vi "Create_Empty_Rx_Channels.vi"(8 "Nb Channels":i32=16, 11 "Rx Channels In":T1[](array[typedef])=[{"Labels Settings"=[{"Name"="label 1", "xmlName"="100", "Label"=23, "transferPeriod"=0, "Driver Data"={"Lbl Tx Hdl"=0, "Decimation"=0, "IterationOffset"=0, "transfer handle"=0, "RX Word"=0, "TXChange"=FALSE, "RX timestamp"=0.0}, "SDI_Enabled"=FALSE, "SDI"=0, "Words"=[{"Block Data Refs"=[], "Values Array"=[0.0], "Length"=1, "FIFO Index"=0, "Param Setting"={"Start Bit"=[10], "Num Bits"=[19], "Signed?"=[FALSE], "ScaleFac"=[1.0], "ScaleOffset"=[0.0], "Channel FIFO Buffer Index"=[1, 0], "Encoding"=[]}}], "bufferSize"=0, "RxWordIdx"=0, "TxWordIdx"=0, "TransferType"=enum."ScheduledLabel", "has timestamp?"=TRUE, "LBL Disable Index"=-1, "Message Handle"=0, "Initialized?"=FALSE}, {"Name"="label 2", "xmlName"="200", "Label"=24, "transferPeriod"=0, "Driver Data"={"Lbl Tx Hdl"=0, "Decimation"=0, "IterationOffset"=0, "transfer handle"=0, "RX Word"=0, "TXChange"=FALSE, "RX timestamp"=0.0}, "SDI_Enabled"=FALSE, "SDI"=0, "Words"=[{"Block Data Refs"=[], "Values Array"=[0.0], "Length"=1, "FIFO Index"=0, "Param Setting"={"Start Bit"=[10], "Num Bits"=[19], "Signed?"=[FALSE], "ScaleFac"=[1.0], "ScaleOffset"=[0.0], "Channel FIFO Buffer Index"=[3, 2], "Encoding"=[]}}], "bufferSize"=0, "RxWordIdx"=0, "TxWordIdx"=0, "TransferType"=enum."ScheduledLabel", "has timestamp?"=TRUE, "LBL Disable Index"=-1, "Message Handle"=0, "Initialized?"=FALSE}, {"Name"="label 3", "xmlName"="300", "Label"=25, "transferPeriod"=0, "Driver Data"={"Lbl Tx Hdl"=0, "Decimation"=0, "IterationOffset"=0, "transfer handle"=0, "RX Word"=0, "TXChange"=FALSE, "RX timestamp"=0.0}, "SDI_Enabled"=FALSE, "SDI"=0, "Words"=[{"Block Data Refs"=[], "Values Array"=[0.0], "Length"=1, "FIFO Index"=0, "Param Setting"={"Start Bit"=[10], "Num Bits"=[19], "Signed?"=[FALSE], "ScaleFac"=[1.0], "ScaleOffset"=[0.0], "Channel FIFO Buffer Index"=[5, 4], "Encoding"=[]}}], "bufferSize"=0, "RxWordIdx"=0, "TxWordIdx"=0, "TransferType"=enum."ScheduledLabel", "has timestamp?"=TRUE, "LBL Disable Index"=-1, "Message Handle"=0, "Initialized?"=FALSE}, {"Name"="label 4", "xmlName"="400", "Label"=26, "transferPeriod"=0, "Driver Data"={"Lbl Tx Hdl"=0, "Decimation"=0, "IterationOffset"=0, "transfer handle"=0, "RX Word"=0, "TXChange"=FALSE, "RX timestamp"=0.0}, "SDI_Enabled"=FALSE, "SDI"=0, "Words"=[{"Block Data Refs"=[], "Values Array"=[0.0], "Length"=1, "FIFO Index"=0, "Param Setting"={"Start Bit"=[10], "Num Bits"=[19], "Signed?"=[FALSE], "ScaleFac"=[1.0], "ScaleOffset"=[0.0], "Channel FIFO Buffer Index"=[7, 6], "Encoding"=[]}}], "bufferSize"=0, "RxWordIdx"=0, "TxWordIdx"=0, "TransferType"=enum."ScheduledLabel", "has timestamp?"=TRUE, "LBL Disable Index"=-1, "Message Handle"=0, "Initialized?"=FALSE}], "channel handle"=0, "channel #"=0, "Label Map"=[], "Label Buffer"=[], "rdBufHandle"=0}, {"Labels Settings"=[{"Name"="label 1", "xmlName"="101", "Label"=23, "transferPeriod"=0, "Driver Data"={"Lbl Tx Hdl"=0, "Decimation"=0, "IterationOffset"=0, "transfer handle"=0, "RX Word"=0, "TXChange"=FALSE, "RX timestamp"=0.0}, "SDI_Enabled"=FALSE, "SDI"=0, "Words"=[{"Block Data Refs"=[], "Values Array"=[0.0], "Length"=1, "FIFO Index"=0, "Param Setting"={"Start Bit"=[10], "Num Bits"=[19], "Signed?"=[FALSE], "ScaleFac"=[1.0], "ScaleOffset"=[0.0], "Channel FIFO Buffer Index"=[9, 8], "Encoding"=[]}}], "bufferSize"=0, "RxWordIdx"=0, "TxWordIdx"=0, "TransferType"=enum."ScheduledLabel", "has timestamp?"=TRUE, "LBL Disable Index"=-1, "Message Handle"=0, "Initialized?"=FALSE}, {"Name"="label 2", "xmlName"="201", "Label"=24, "transferPeriod"=0, "Driver Data"={"Lbl Tx Hdl"=0, "Decimation"=0, "IterationOffset"=0, "transfer handle"=0, "RX Word"=0, "TXChange"=FALSE, "RX timestamp"=0.0}, "SDI_Enabled"=FALSE, "SDI"=0, "Words"=[{"Block Data Refs"=[], "Values Array"=[0.0], "Length"=1, "FIFO Index"=0, "Param Setting"={"Start Bit"=[10], "Num Bits"=[19], "Signed?"=[FALSE], "ScaleFac"=[1.0], "ScaleOffset"=[0.0], "Channel FIFO Buffer Index"=[11, 10], "Encoding"=[]}}], "bufferSize"=0, "RxWordIdx"=0, "TxWordIdx"=0, "TransferType"=enum."ScheduledLabel", "has timestamp?"=TRUE, "LBL Disable Index"=-1, "Message Handle"=0, "Initialized?"=FALSE}, {"Name"="label 3", "xmlName"="301", "Label"=25, "transferPeriod"=0, "Driver Data"={"Lbl Tx Hdl"=0, "Decimation"=0, "IterationOffset"=0, "transfer handle"=0, "RX Word"=0, "TXChange"=FALSE, "RX timestamp"=0.0}, "SDI_Enabled"=FALSE, "SDI"=0, "Words"=[{"Block Data Refs"=[], "Values Array"=[0.0], "Length"=1, "FIFO Index"=0, "Param Setting"={"Start Bit"=[10], "Num Bits"=[19], "Signed?"=[FALSE], "ScaleFac"=[1.0], "ScaleOffset"=[0.0], "Channel FIFO Buffer Index"=[13, 12], "Encoding"=[]}}], "bufferSize"=0, "RxWordIdx"=0, "TxWordIdx"=0, "TransferType"=enum."ScheduledLabel", "has timestamp?"=TRUE, "LBL Disable Index"=-1, "Message Handle"=0, "Initialized?"=FALSE}, {"Name"="label 4", "xmlName"="401", "Label"=26, "transferPeriod"=0, "Driver Data"={"Lbl Tx Hdl"=0, "Decimation"=0, "IterationOffset"=0, "transfer handle"=0, "RX Word"=0, "TXChange"=FALSE, "RX timestamp"=0.0}, "SDI_Enabled"=FALSE, "SDI"=0, "Words"=[{"Block Data Refs"=[], "Values Array"=[0.0], "Length"=1, "FIFO Index"=0, "Param Setting"={"Start Bit"=[10], "Num Bits"=[19], "Signed?"=[FALSE], "ScaleFac"=[1.0], "ScaleOffset"=[0.0], "Channel FIFO Buffer Index"=[15, 14], "Encoding"=[]}}], "bufferSize"=0, "RxWordIdx"=0, "TxWordIdx"=0, "TransferType"=enum."ScheduledLabel", "has timestamp?"=TRUE, "LBL Disable Index"=-1, "Message Handle"=0, "Initialized?"=FALSE}, {"Name"="label 5", "xmlName"="501", "Label"=27, "transferPeriod"=0, "Driver Data"={"Lbl Tx Hdl"=0, "Decimation"=0, "IterationOffset"=0, "transfer handle"=0, "RX Word"=0, "TXChange"=FALSE, "RX timestamp"=0.0}, "SDI_Enabled"=FALSE, "SDI"=0, "Words"=[{"Block Data Refs"=[], "Values Array"=[0.0], "Length"=1, "FIFO Index"=0, "Param Setting"={"Start Bit"=[10], "Num Bits"=[19], "Signed?"=[FALSE], "ScaleFac"=[1.0], "ScaleOffset"=[0.0], "Channel FIFO Buffer Index"=[17, 16], "Encoding"=[]}}], "bufferSize"=0, "RxWordIdx"=0, "TxWordIdx"=0, "TransferType"=enum."ScheduledLabel", "has timestamp?"=TRUE, "LBL Disable Index"=-1, "Message Handle"=0, "Initialized?"=FALSE}, {"Name"="label 6", "xmlName"="601", "Label"=28, "transferPeriod"=0, "Driver Data"={"Lbl Tx Hdl"=0, "Decimation"=0, "IterationOffset"=0, "transfer handle"=0, "RX Word"=0, "TXChange"=FALSE, "RX timestamp"=0.0}, "SDI_Enabled"=FALSE, "SDI"=0, "Words"=[{"Block Data Refs"=[], "Values Array"=[0.0], "Length"=1, "FIFO Index"=0, "Param Setting"={"Start Bit"=[10], "Num Bits"=[19], "Signed?"=[FALSE], "ScaleFac"=[1.0], "ScaleOffset"=[0.0], "Channel FIFO Buffer Index"=[19, 18], "Encoding"=[]}}], "bufferSize"=0, "RxWordIdx"=0, "TxWordIdx"=0, "TransferType"=enum."ScheduledLabel", "has timestamp?"=TRUE, "LBL Disable Index"=-1, "Message Handle"=0, "Initialized?"=FALSE}], "channel handle"=0, "channel #"=1, "Label Map"=[], "Label Buffer"=[], "rdBufHandle"=0}, {"Labels Settings"=[{"Name"="label 1", "xmlName"="102", "Label"=23, "transferPeriod"=0, "Driver Data"={"Lbl Tx Hdl"=0, "Decimation"=0, "IterationOffset"=0, "transfer handle"=0, "RX Word"=0, "TXChange"=FALSE, "RX timestamp"=0.0}, "SDI_Enabled"=FALSE, "SDI"=0, "Words"=[{"Block Data Refs"=[], "Values Array"=[0.0], "Length"=1, "FIFO Index"=0, "Param Setting"={"Start Bit"=[10], "Num Bits"=[19], "Signed?"=[FALSE], "ScaleFac"=[1.0], "ScaleOffset"=[0.0], "Channel FIFO Buffer Index"=[21, 20], "Encoding"=[]}}], "bufferSize"=0, "RxWordIdx"=0, "TxWordIdx"=0, "TransferType"=enum."ScheduledLabel", "has timestamp?"=TRUE, "LBL Disable Index"=-1, "Message Handle"=0, "Initialized?"=FALSE}, {"Name"="label 2", "xmlName"="202", "Label"=24, "transferPeriod"=0, "Driver Data"={"Lbl Tx Hdl"=0, "Decimation"=0, "IterationOffset"=0, "transfer handle"=0, "RX Word"=0, "TXChange"=FALSE, "RX timestamp"=0.0}, "SDI_Enabled"=FALSE, "SDI"=0, "Words"=[{"Block Data Refs"=[], "Values Array"=[0.0], "Length"=1, "FIFO Index"=0, "Param Setting"={"Start Bit"=[10], "Num Bits"=[19], "Signed?"=[FALSE], "ScaleFac"=[1.0], "ScaleOffset"=[0.0], "Channel FIFO Buffer Index"=[23, 22], "Encoding"=[]}}], "bufferSize"=0, "RxWordIdx"=0, "TxWordIdx"=0, "TransferType"=enum."ScheduledLabel", "has timestamp?"=TRUE, "LBL Disable Index"=-1, "Message Handle"=0, "Initialized?"=FALSE}, {"Name"="label 3", "xmlName"="302", "Label"=25, "transferPeriod"=0, "Driver Data"={"Lbl Tx Hdl"=0, "Decimation"=0, "IterationOffset"=0, "transfer handle"=0, "RX Word"=0, "TXChange"=FALSE, "RX timestamp"=0.0}, "SDI_Enabled"=FALSE, "SDI"=0, "Words"=[{"Block Data Refs"=[], "Values Array"=[0.0], "Length"=1, "FIFO Index"=0, "Param Setting"={"Start Bit"=[10], "Num Bits"=[19], "Signed?"=[FALSE], "ScaleFac"=[1.0], "ScaleOffset"=[0.0], "Channel FIFO Buffer Index"=[25, 24], "Encoding"=[]}}], "bufferSize"=0, "RxWordIdx"=0, "TxWordIdx"=0, "TransferType"=enum."ScheduledLabel", "has timestamp?"=TRUE, "LBL Disable Index"=-1, "Message Handle"=0, "Initialized?"=FALSE}, {"Name"="label 4", "xmlName"="402", "Label"=26, "transferPeriod"=0, "Driver Data"={"Lbl Tx Hdl"=0, "Decimation"=0, "IterationOffset"=0, "transfer handle"=0, "RX Word"=0, "TXChange"=FALSE, "RX timestamp"=0.0}, "SDI_Enabled"=FALSE, "SDI"=0, "Words"=[{"Block Data Refs"=[], "Values Array"=[0.0], "Length"=1, "FIFO Index"=0, "Param Setting"={"Start Bit"=[10], "Num Bits"=[19], "Signed?"=[FALSE], "ScaleFac"=[1.0], "ScaleOffset"=[0.0], "Channel FIFO Buffer Index"=[27, 26], "Encoding"=[]}}], "bufferSize"=0, "RxWordIdx"=0, "TxWordIdx"=0, "TransferType"=enum."ScheduledLabel", "has timestamp?"=TRUE, "LBL Disable Index"=-1, "Message Handle"=0, "Initialized?"=FALSE}, {"Name"="label 5", "xmlName"="502", "Label"=27, "transferPeriod"=0, "Driver Data"={"Lbl Tx Hdl"=0, "Decimation"=0, "IterationOffset"=0, "transfer handle"=0, "RX Word"=0, "TXChange"=FALSE, "RX timestamp"=0.0}, "SDI_Enabled"=FALSE, "SDI"=0, "Words"=[{"Block Data Refs"=[], "Values Array"=[0.0], "Length"=1, "FIFO Index"=0, "Param Setting"={"Start Bit"=[10], "Num Bits"=[19], "Signed?"=[FALSE], "ScaleFac"=[1.0], "ScaleOffset"=[0.0], "Channel FIFO Buffer Index"=[28, 29], "Encoding"=[]}}], "bufferSize"=0, "RxWordIdx"=0, "TxWordIdx"=0, "TransferType"=enum."ScheduledLabel", "has timestamp?"=TRUE, "LBL Disable Index"=-1, "Message Handle"=0, "Initialized?"=FALSE}, {"Name"="label 6", "xmlName"="602", "Label"=28, "transferPeriod"=0, "Driver Data"={"Lbl Tx Hdl"=0, "Decimation"=0, "IterationOffset"=0, "transfer handle"=0, "RX Word"=0, "TXChange"=FALSE, "RX timestamp"=0.0}, "SDI_Enabled"=FALSE, "SDI"=0, "Words"=[{"Block Data Refs"=[], "Values Array"=[0.0], "Length"=1, "FIFO Index"=0, "Param Setting"={"Start Bit"=[10], "Num Bits"=[19], "Signed?"=[FALSE], "ScaleFac"=[1.0], "ScaleOffset"=[0.0], "Channel FIFO Buffer Index"=[31, 30], "Encoding"=[]}}], "bufferSize"=0, "RxWordIdx"=0, "TxWordIdx"=0, "TransferType"=enum."ScheduledLabel", "has timestamp?"=TRUE, "LBL Disable Index"=-1, "Message Handle"=0, "Initialized?"=FALSE}, {"Name"="label 7", "xmlName"="702", "Label"=29, "transferPeriod"=0, "Driver Data"={"Lbl Tx Hdl"=0, "Decimation"=0, "IterationOffset"=0, "transfer handle"=0, "RX Word"=0, "TXChange"=FALSE, "RX timestamp"=0.0}, "SDI_Enabled"=FALSE, "SDI"=0, "Words"=[{"Block Data Refs"=[], "Values Array"=[0.0], "Length"=1, "FIFO Index"=0, "Param Setting"={"Start Bit"=[10], "Num Bits"=[19], "Signed?"=[FALSE], "ScaleFac"=[1.0], "ScaleOffset"=[0.0], "Channel FIFO Buffer Index"=[33, 32], "Encoding"=[]}}], "bufferSize"=0, "RxWordIdx"=0, "TxWordIdx"=0, "TransferType"=enum."ScheduledLabel", "has timestamp?"=TRUE, "LBL Disable Index"=-1, "Message Handle"=0, "Initialized?"=FALSE}, {"Name"="label 8", "xmlName"="802", "Label"=30, "transferPeriod"=0, "Driver Data"={"Lbl Tx Hdl"=0, "Decimation"=0, "IterationOffset"=0, "transfer handle"=0, "RX Word"=0, "TXChange"=FALSE, "RX timestamp"=0.0}, "SDI_Enabled"=FALSE, "SDI"=0, "Words"=[{"Block Data Refs"=[], "Values Array"=[0.0], "Length"=1, "FIFO Index"=0, "Param Setting"={"Start Bit"=[10], "Num Bits"=[19], "Signed?"=[FALSE], "ScaleFac"=[1.0], "ScaleOffset"=[0.0], "Channel FIFO Buffer Index"=[35, 34], "Encoding"=[]}}], "bufferSize"=0, "RxWordIdx"=0, "TxWordIdx"=0, "TransferType"=enum."ScheduledLabel", "has timestamp?"=TRUE, "LBL Disable Index"=-1, "Message Handle"=0, "Initialized?"=FALSE}], "channel handle"=0, "channel #"=2, "Label Map"=[], "Label Buffer"=[], "rdBufHandle"=0}, {"Labels Settings"=[{"Name"="label 1 SDI 01", "xmlName"="10301", "Label"=23, "transferPeriod"=0, "Driver Data"={"Lbl Tx Hdl"=0, "Decimation"=0, "IterationOffset"=0, "transfer handle"=0, "RX Word"=0, "TXChange"=FALSE, "RX timestamp"=0.0}, "SDI_Enabled"=TRUE, "SDI"=1, "Words"=[{"Block Data Refs"=[], "Values Array"=[0.0], "Length"=1, "FIFO Index"=0, "Param Setting"={"Start Bit"=[10], "Num Bits"=[19], "Signed?"=[FALSE], "ScaleFac"=[1.0], "ScaleOffset"=[0.0], "Channel FIFO Buffer Index"=[37, 36], "Encoding"=[]}}], "bufferSize"=0, "RxWordIdx"=0, "TxWordIdx"=0, "TransferType"=enum."ScheduledLabel", "has timestamp?"=TRUE, "LBL Disable Index"=-1, "Message Handle"=0, "Initialized?"=FALSE}, {"Name"="label 1 SDI 10", "xmlName"="10310", "Label"=23, "transferPeriod"=0, "Driver Data"={"Lbl Tx Hdl"=0, "Decimation"=0, "IterationOffset"=0, "transfer handle"=0, "RX Word"=0, "TXChange"=FALSE, "RX timestamp"=0.0}, "SDI_Enabled"=TRUE, "SDI"=10, "Words"=[{"Block Data Refs"=[], "Values Array"=[0.0], "Length"=1, "FIFO Index"=0, "Param Setting"={"Start Bit"=[10], "Num Bits"=[19], "Signed?"=[FALSE], "ScaleFac"=[1.0], "ScaleOffset"=[0.0], "Channel FIFO Buffer Index"=[39, 38], "Encoding"=[]}}], "bufferSize"=0, "RxWordIdx"=0, "TxWordIdx"=0, "TransferType"=enum."ScheduledLabel", "has timestamp?"=TRUE, "LBL Disable Index"=-1, "Message Handle"=0, "Initialized?"=FALSE}, {"Name"="label 2", "xmlName"="203", "Label"=24, "transferPeriod"=0, "Driver Data"={"Lbl Tx Hdl"=0, "Decimation"=0, "IterationOffset"=0, "transfer handle"=0, "RX Word"=0, "TXChange"=FALSE, "RX timestamp"=0.0}, "SDI_Enabled"=FALSE, "SDI"=0, "Words"=[{"Block Data Refs"=[], "Values Array"=[0.0], "Length"=1, "FIFO Index"=0, "Param Setting"={"Start Bit"=[10], "Num Bits"=[19], "Signed?"=[FALSE], "ScaleFac"=[1.0], "ScaleOffset"=[0.0], "Channel FIFO Buffer Index"=[41, 40], "Encoding"=[]}}], "bufferSize"=0, "RxWordIdx"=0, "TxWordIdx"=0, "TransferType"=enum."ScheduledLabel", "has timestamp?"=TRUE, "LBL Disable Index"=-1, "Message Handle"=0, "Initialized?"=FALSE}], "channel handle"=0, "channel #"=3, "Label Map"=[], "Label Buffer"=[], "rdBufHandle"=0}] {"Labels Settings"."Label" format="%.0o"}) -> (3 "Rx Channels Out":T1[](array[typedef])=[{"Labels Settings"=[{"Name"="label 1", "xmlName"="100", "Label"=23, "transferPeriod"=0, "Driver Data"={"Lbl Tx Hdl"=0, "Decimation"=0, "IterationOffset"=0, "transfer handle"=0, "RX Word"=0, "TXChange"=FALSE, "RX timestamp"=0.0}, "SDI_Enabled"=FALSE, "SDI"=0, "Words"=[{"Block Data Refs"=[], "Values Array"=[0.0], "Length"=1, "FIFO Index"=0, "Param Setting"={"Start Bit"=[10], "Num Bits"=[19], "Signed?"=[FALSE], "ScaleFac"=[1.0], "ScaleOffset"=[0.0], "Channel FIFO Buffer Index"=[1, 0], "Encoding"=[]}}], "bufferSize"=0, "RxWordIdx"=0, "TxWordIdx"=0, "TransferType"=enum."ScheduledLabel", "has timestamp?"=TRUE, "LBL Disable Index"=-1, "Message Handle"=0, "Initialized?"=FALSE}, {"Name"="label 2", "xmlName"="200", "Label"=24, "transferPeriod"=0, "Driver Data"={"Lbl Tx Hdl"=0, "Decimation"=0, "IterationOffset"=0, "transfer handle"=0, "RX Word"=0, "TXChange"=FALSE, "RX timestamp"=0.0}, "SDI_Enabled"=FALSE, "SDI"=0, "Words"=[{"Block Data Refs"=[], "Values Array"=[0.0], "Length"=1, "FIFO Index"=0, "Param Setting"={"Start Bit"=[10], "Num Bits"=[19], "Signed?"=[FALSE], "ScaleFac"=[1.0], "ScaleOffset"=[0.0], "Channel FIFO Buffer Index"=[3, 2], "Encoding"=[]}}], "bufferSize"=0, "RxWordIdx"=0, "TxWordIdx"=0, "TransferType"=enum."ScheduledLabel", "has timestamp?"=TRUE, "LBL Disable Index"=-1, "Message Handle"=0, "Initialized?"=FALSE}, {"Name"="label 3", "xmlName"="300", "Label"=25, "transferPeriod"=0, "Driver Data"={"Lbl Tx Hdl"=0, "Decimation"=0, "IterationOffset"=0, "transfer handle"=0, "RX Word"=0, "TXChange"=FALSE, "RX timestamp"=0.0}, "SDI_Enabled"=FALSE, "SDI"=0, "Words"=[{"Block Data Refs"=[], "Values Array"=[0.0], "Length"=1, "FIFO Index"=0, "Param Setting"={"Start Bit"=[10], "Num Bits"=[19], "Signed?"=[FALSE], "ScaleFac"=[1.0], "ScaleOffset"=[0.0], "Channel FIFO Buffer Index"=[5, 4], "Encoding"=[]}}], "bufferSize"=0, "RxWordIdx"=0, "TxWordIdx"=0, "TransferType"=enum."ScheduledLabel", "has timestamp?"=TRUE, "LBL Disable Index"=-1, "Message Handle"=0, "Initialized?"=FALSE}, {"Name"="label 4", "xmlName"="400", "Label"=26, "transferPeriod"=0, "Driver Data"={"Lbl Tx Hdl"=0, "Decimation"=0, "IterationOffset"=0, "transfer handle"=0, "RX Word"=0, "TXChange"=FALSE, "RX timestamp"=0.0}, "SDI_Enabled"=FALSE, "SDI"=0, "Words"=[{"Block Data Refs"=[], "Values Array"=[0.0], "Length"=1, "FIFO Index"=0, "Param Setting"={"Start Bit"=[10], "Num Bits"=[19], "Signed?"=[FALSE], "ScaleFac"=[1.0], "ScaleOffset"=[0.0], "Channel FIFO Buffer Index"=[7, 6], "Encoding"=[]}}], "bufferSize"=0, "RxWordIdx"=0, "TxWordIdx"=0, "TransferType"=enum."ScheduledLabel", "has timestamp?"=TRUE, "LBL Disable Index"=-1, "Message Handle"=0, "Initialized?"=FALSE}], "channel handle"=0, "channel #"=0, "Label Map"=[], "Label Buffer"=[], "rdBufHandle"=0}, {"Labels Settings"=[{"Name"="label 1", "xmlName"="101", "Label"=23, "transferPeriod"=0, "Driver Data"={"Lbl Tx Hdl"=0, "Decimation"=0, "IterationOffset"=0, "transfer handle"=0, "RX Word"=0, "TXChange"=FALSE, "RX timestamp"=0.0}, "SDI_Enabled"=FALSE, "SDI"=0, "Words"=[{"Block Data Refs"=[], "Values Array"=[0.0], "Length"=1, "FIFO Index"=0, "Param Setting"={"Start Bit"=[10], "Num Bits"=[19], "Signed?"=[FALSE], "ScaleFac"=[1.0], "ScaleOffset"=[0.0], "Channel FIFO Buffer Index"=[9, 8], "Encoding"=[]}}], "bufferSize"=0, "RxWordIdx"=0, "TxWordIdx"=0, "TransferType"=enum."ScheduledLabel", "has timestamp?"=TRUE, "LBL Disable Index"=-1, "Message Handle"=0, "Initialized?"=FALSE}, {"Name"="label 2", "xmlName"="201", "Label"=24, "transferPeriod"=0, "Driver Data"={"Lbl Tx Hdl"=0, "Decimation"=0, "IterationOffset"=0, "transfer handle"=0, "RX Word"=0, "TXChange"=FALSE, "RX timestamp"=0.0}, "SDI_Enabled"=FALSE, "SDI"=0, "Words"=[{"Block Data Refs"=[], "Values Array"=[0.0], "Length"=1, "FIFO Index"=0, "Param Setting"={"Start Bit"=[10], "Num Bits"=[19], "Signed?"=[FALSE], "ScaleFac"=[1.0], "ScaleOffset"=[0.0], "Channel FIFO Buffer Index"=[11, 10], "Encoding"=[]}}], "bufferSize"=0, "RxWordIdx"=0, "TxWordIdx"=0, "TransferType"=enum."ScheduledLabel", "has timestamp?"=TRUE, "LBL Disable Index"=-1, "Message Handle"=0, "Initialized?"=FALSE}, {"Name"="label 3", "xmlName"="301", "Label"=25, "transferPeriod"=0, "Driver Data"={"Lbl Tx Hdl"=0, "Decimation"=0, "IterationOffset"=0, "transfer handle"=0, "RX Word"=0, "TXChange"=FALSE, "RX timestamp"=0.0}, "SDI_Enabled"=FALSE, "SDI"=0, "Words"=[{"Block Data Refs"=[], "Values Array"=[0.0], "Length"=1, "FIFO Index"=0, "Param Setting"={"Start Bit"=[10], "Num Bits"=[19], "Signed?"=[FALSE], "ScaleFac"=[1.0], "ScaleOffset"=[0.0], "Channel FIFO Buffer Index"=[13, 12], "Encoding"=[]}}], "bufferSize"=0, "RxWordIdx"=0, "TxWordIdx"=0, "TransferType"=enum."ScheduledLabel", "has timestamp?"=TRUE, "LBL Disable Index"=-1, "Message Handle"=0, "Initialized?"=FALSE}, {"Name"="label 4", "xmlName"="401", "Label"=26, "transferPeriod"=0, "Driver Data"={"Lbl Tx Hdl"=0, "Decimation"=0, "IterationOffset"=0, "transfer handle"=0, "RX Word"=0, "TXChange"=FALSE, "RX timestamp"=0.0}, "SDI_Enabled"=FALSE, "SDI"=0, "Words"=[{"Block Data Refs"=[], "Values Array"=[0.0], "Length"=1, "FIFO Index"=0, "Param Setting"={"Start Bit"=[10], "Num Bits"=[19], "Signed?"=[FALSE], "ScaleFac"=[1.0], "ScaleOffset"=[0.0], "Channel FIFO Buffer Index"=[15, 14], "Encoding"=[]}}], "bufferSize"=0, "RxWordIdx"=0, "TxWordIdx"=0, "TransferType"=enum."ScheduledLabel", "has timestamp?"=TRUE, "LBL Disable Index"=-1, "Message Handle"=0, "Initialized?"=FALSE}, {"Name"="label 5", "xmlName"="501", "Label"=27, "transferPeriod"=0, "Driver Data"={"Lbl Tx Hdl"=0, "Decimation"=0, "IterationOffset"=0, "transfer handle"=0, "RX Word"=0, "TXChange"=FALSE, "RX timestamp"=0.0}, "SDI_Enabled"=FALSE, "SDI"=0, "Words"=[{"Block Data Refs"=[], "Values Array"=[0.0], "Length"=1, "FIFO Index"=0, "Param Setting"={"Start Bit"=[10], "Num Bits"=[19], "Signed?"=[FALSE], "ScaleFac"=[1.0], "ScaleOffset"=[0.0], "Channel FIFO Buffer Index"=[17, 16], "Encoding"=[]}}], "bufferSize"=0, "RxWordIdx"=0, "TxWordIdx"=0, "TransferType"=enum."ScheduledLabel", "has timestamp?"=TRUE, "LBL Disable Index"=-1, "Message Handle"=0, "Initialized?"=FALSE}, {"Name"="label 6", "xmlName"="601", "Label"=28, "transferPeriod"=0, "Driver Data"={"Lbl Tx Hdl"=0, "Decimation"=0, "IterationOffset"=0, "transfer handle"=0, "RX Word"=0, "TXChange"=FALSE, "RX timestamp"=0.0}, "SDI_Enabled"=FALSE, "SDI"=0, "Words"=[{"Block Data Refs"=[], "Values Array"=[0.0], "Length"=1, "FIFO Index"=0, "Param Setting"={"Start Bit"=[10], "Num Bits"=[19], "Signed?"=[FALSE], "ScaleFac"=[1.0], "ScaleOffset"=[0.0], "Channel FIFO Buffer Index"=[19, 18], "Encoding"=[]}}], "bufferSize"=0, "RxWordIdx"=0, "TxWordIdx"=0, "TransferType"=enum."ScheduledLabel", "has timestamp?"=TRUE, "LBL Disable Index"=-1, "Message Handle"=0, "Initialized?"=FALSE}], "channel handle"=0, "channel #"=1, "Label Map"=[], "Label Buffer"=[], "rdBufHandle"=0}, {"Labels Settings"=[{"Name"="label 1", "xmlName"="102", "Label"=23, "transferPeriod"=0, "Driver Data"={"Lbl Tx Hdl"=0, "Decimation"=0, "IterationOffset"=0, "transfer handle"=0, "RX Word"=0, "TXChange"=FALSE, "RX timestamp"=0.0}, "SDI_Enabled"=FALSE, "SDI"=0, "Words"=[{"Block Data Refs"=[], "Values Array"=[0.0], "Length"=1, "FIFO Index"=0, "Param Setting"={"Start Bit"=[10], "Num Bits"=[19], "Signed?"=[FALSE], "ScaleFac"=[1.0], "ScaleOffset"=[0.0], "Channel FIFO Buffer Index"=[21, 20], "Encoding"=[]}}], "bufferSize"=0, "RxWordIdx"=0, "TxWordIdx"=0, "TransferType"=enum."ScheduledLabel", "has timestamp?"=TRUE, "LBL Disable Index"=-1, "Message Handle"=0, "Initialized?"=FALSE}, {"Name"="label 2", "xmlName"="202", "Label"=24, "transferPeriod"=0, "Driver Data"={"Lbl Tx Hdl"=0, "Decimation"=0, "IterationOffset"=0, "transfer handle"=0, "RX Word"=0, "TXChange"=FALSE, "RX timestamp"=0.0}, "SDI_Enabled"=FALSE, "SDI"=0, "Words"=[{"Block Data Refs"=[], "Values Array"=[0.0], "Length"=1, "FIFO Index"=0, "Param Setting"={"Start Bit"=[10], "Num Bits"=[19], "Signed?"=[FALSE], "ScaleFac"=[1.0], "ScaleOffset"=[0.0], "Channel FIFO Buffer Index"=[23, 22], "Encoding"=[]}}], "bufferSize"=0, "RxWordIdx"=0, "TxWordIdx"=0, "TransferType"=enum."ScheduledLabel", "has timestamp?"=TRUE, "LBL Disable Index"=-1, "Message Handle"=0, "Initialized?"=FALSE}, {"Name"="label 3", "xmlName"="302", "Label"=25, "transferPeriod"=0, "Driver Data"={"Lbl Tx Hdl"=0, "Decimation"=0, "IterationOffset"=0, "transfer handle"=0, "RX Word"=0, "TXChange"=FALSE, "RX timestamp"=0.0}, "SDI_Enabled"=FALSE, "SDI"=0, "Words"=[{"Block Data Refs"=[], "Values Array"=[0.0], "Length"=1, "FIFO Index"=0, "Param Setting"={"Start Bit"=[10], "Num Bits"=[19], "Signed?"=[FALSE], "ScaleFac"=[1.0], "ScaleOffset"=[0.0], "Channel FIFO Buffer Index"=[25, 24], "Encoding"=[]}}], "bufferSize"=0, "RxWordIdx"=0, "TxWordIdx"=0, "TransferType"=enum."ScheduledLabel", "has timestamp?"=TRUE, "LBL Disable Index"=-1, "Message Handle"=0, "Initialized?"=FALSE}, {"Name"="label 4", "xmlName"="402", "Label"=26, "transferPeriod"=0, "Driver Data"={"Lbl Tx Hdl"=0, "Decimation"=0, "IterationOffset"=0, "transfer handle"=0, "RX Word"=0, "TXChange"=FALSE, "RX timestamp"=0.0}, "SDI_Enabled"=FALSE, "SDI"=0, "Words"=[{"Block Data Refs"=[], "Values Array"=[0.0], "Length"=1, "FIFO Index"=0, "Param Setting"={"Start Bit"=[10], "Num Bits"=[19], "Signed?"=[FALSE], "ScaleFac"=[1.0], "ScaleOffset"=[0.0], "Channel FIFO Buffer Index"=[27, 26], "Encoding"=[]}}], "bufferSize"=0, "RxWordIdx"=0, "TxWordIdx"=0, "TransferType"=enum."ScheduledLabel", "has timestamp?"=TRUE, "LBL Disable Index"=-1, "Message Handle"=0, "Initialized?"=FALSE}, {"Name"="label 5", "xmlName"="502", "Label"=27, "transferPeriod"=0, "Driver Data"={"Lbl Tx Hdl"=0, "Decimation"=0, "IterationOffset"=0, "transfer handle"=0, "RX Word"=0, "TXChange"=FALSE, "RX timestamp"=0.0}, "SDI_Enabled"=FALSE, "SDI"=0, "Words"=[{"Block Data Refs"=[], "Values Array"=[0.0], "Length"=1, "FIFO Index"=0, "Param Setting"={"Start Bit"=[10], "Num Bits"=[19], "Signed?"=[FALSE], "ScaleFac"=[1.0], "ScaleOffset"=[0.0], "Channel FIFO Buffer Index"=[28, 29], "Encoding"=[]}}], "bufferSize"=0, "RxWordIdx"=0, "TxWordIdx"=0, "TransferType"=enum."ScheduledLabel", "has timestamp?"=TRUE, "LBL Disable Index"=-1, "Message Handle"=0, "Initialized?"=FALSE}, {"Name"="label 6", "xmlName"="602", "Label"=28, "transferPeriod"=0, "Driver Data"={"Lbl Tx Hdl"=0, "Decimation"=0, "IterationOffset"=0, "transfer handle"=0, "RX Word"=0, "TXChange"=FALSE, "RX timestamp"=0.0}, "SDI_Enabled"=FALSE, "SDI"=0, "Words"=[{"Block Data Refs"=[], "Values Array"=[0.0], "Length"=1, "FIFO Index"=0, "Param Setting"={"Start Bit"=[10], "Num Bits"=[19], "Signed?"=[FALSE], "ScaleFac"=[1.0], "ScaleOffset"=[0.0], "Channel FIFO Buffer Index"=[31, 30], "Encoding"=[]}}], "bufferSize"=0, "RxWordIdx"=0, "TxWordIdx"=0, "TransferType"=enum."ScheduledLabel", "has timestamp?"=TRUE, "LBL Disable Index"=-1, "Message Handle"=0, "Initialized?"=FALSE}, {"Name"="label 7", "xmlName"="702", "Label"=29, "transferPeriod"=0, "Driver Data"={"Lbl Tx Hdl"=0, "Decimation"=0, "IterationOffset"=0, "transfer handle"=0, "RX Word"=0, "TXChange"=FALSE, "RX timestamp"=0.0}, "SDI_Enabled"=FALSE, "SDI"=0, "Words"=[{"Block Data Refs"=[], "Values Array"=[0.0], "Length"=1, "FIFO Index"=0, "Param Setting"={"Start Bit"=[10], "Num Bits"=[19], "Signed?"=[FALSE], "ScaleFac"=[1.0], "ScaleOffset"=[0.0], "Channel FIFO Buffer Index"=[33, 32], "Encoding"=[]}}], "bufferSize"=0, "RxWordIdx"=0, "TxWordIdx"=0, "TransferType"=enum."ScheduledLabel", "has timestamp?"=TRUE, "LBL Disable Index"=-1, "Message Handle"=0, "Initialized?"=FALSE}, {"Name"="label 8", "xmlName"="802", "Label"=30, "transferPeriod"=0, "Driver Data"={"Lbl Tx Hdl"=0, "Decimation"=0, "IterationOffset"=0, "transfer handle"=0, "RX Word"=0, "TXChange"=FALSE, "RX timestamp"=0.0}, "SDI_Enabled"=FALSE, "SDI"=0, "Words"=[{"Block Data Refs"=[], "Values Array"=[0.0], "Length"=1, "FIFO Index"=0, "Param Setting"={"Start Bit"=[10], "Num Bits"=[19], "Signed?"=[FALSE], "ScaleFac"=[1.0], "ScaleOffset"=[0.0], "Channel FIFO Buffer Index"=[35, 34], "Encoding"=[]}}], "bufferSize"=0, "RxWordIdx"=0, "TxWordIdx"=0, "TransferType"=enum."ScheduledLabel", "has timestamp?"=TRUE, "LBL Disable Index"=-1, "Message Handle"=0, "Initialized?"=FALSE}], "channel handle"=0, "channel #"=2, "Label Map"=[], "Label Buffer"=[], "rdBufHandle"=0}, {"Labels Settings"=[{"Name"="label 1 SDI 01", "xmlName"="10301", "Label"=23, "transferPeriod"=0, "Driver Data"={"Lbl Tx Hdl"=0, "Decimation"=0, "IterationOffset"=0, "transfer handle"=0, "RX Word"=0, "TXChange"=FALSE, "RX timestamp"=0.0}, "SDI_Enabled"=TRUE, "SDI"=1, "Words"=[{"Block Data Refs"=[], "Values Array"=[0.0], "Length"=1, "FIFO Index"=0, "Param Setting"={"Start Bit"=[10], "Num Bits"=[19], "Signed?"=[FALSE], "ScaleFac"=[1.0], "ScaleOffset"=[0.0], "Channel FIFO Buffer Index"=[37, 36], "Encoding"=[]}}], "bufferSize"=0, "RxWordIdx"=0, "TxWordIdx"=0, "TransferType"=enum."ScheduledLabel", "has timestamp?"=TRUE, "LBL Disable Index"=-1, "Message Handle"=0, "Initialized?"=FALSE}, {"Name"="label 1 SDI 10", "xmlName"="10310", "Label"=23, "transferPeriod"=0, "Driver Data"={"Lbl Tx Hdl"=0, "Decimation"=0, "IterationOffset"=0, "transfer handle"=0, "RX Word"=0, "TXChange"=FALSE, "RX timestamp"=0.0}, "SDI_Enabled"=TRUE, "SDI"=10, "Words"=[{"Block Data Refs"=[], "Values Array"=[0.0], "Length"=1, "FIFO Index"=0, "Param Setting"={"Start Bit"=[10], "Num Bits"=[19], "Signed?"=[FALSE], "ScaleFac"=[1.0], "ScaleOffset"=[0.0], "Channel FIFO Buffer Index"=[39, 38], "Encoding"=[]}}], "bufferSize"=0, "RxWordIdx"=0, "TxWordIdx"=0, "TransferType"=enum."ScheduledLabel", "has timestamp?"=TRUE, "LBL Disable Index"=-1, "Message Handle"=0, "Initialized?"=FALSE}, {"Name"="label 2", "xmlName"="203", "Label"=24, "transferPeriod"=0, "Driver Data"={"Lbl Tx Hdl"=0, "Decimation"=0, "IterationOffset"=0, "transfer handle"=0, "RX Word"=0, "TXChange"=FALSE, "RX timestamp"=0.0}, "SDI_Enabled"=FALSE, "SDI"=0, "Words"=[{"Block Data Refs"=[], "Values Array"=[0.0], "Length"=1, "FIFO Index"=0, "Param Setting"={"Start Bit"=[10], "Num Bits"=[19], "Signed?"=[FALSE], "ScaleFac"=[1.0], "ScaleOffset"=[0.0], "Channel FIFO Buffer Index"=[41, 40], "Encoding"=[]}}], "bufferSize"=0, "RxWordIdx"=0, "TxWordIdx"=0, "TransferType"=enum."ScheduledLabel", "has timestamp?"=TRUE, "LBL Disable Index"=-1, "Message Handle"=0, "Initialized?"=FALSE}], "channel handle"=0, "channel #"=3, "Label Map"=[], "Label Buffer"=[], "rdBufHandle"=0}] {"Labels Settings"."Label" format="%.0o"})   [LabVIEW 2017, in "Ballard Arinc-429 Engine.lvlib"]
uses:
  Ballard Arinc-429 Engine.lvlib
  RT Controls/RT HW Channel.ctl
  RT Controls/RT Label Settings.ctl
  Shared/Controls and Global/Label.ctl
  Shared/Controls and Global/transferPeriod.ctl
  RT Controls/Driver Data.ctl
  RT Controls/RT Word Settings.ctl
  <vilib>/NI Veristand/Custom Device API/Block Data Reference.ctl
  <vilib>/NI Veristand/Custom Device API/Data Reference.ctl
  RT Controls/RT Param Setting.ctl
  Shared/Controls and Global/Start Bit.ctl
  Shared/Controls and Global/Number of Bits.ctl
  Shared/Controls and Global/TransferType.ctl
  Shared/Ballard Arinc-429 Shared.lvlib
  <vilib>/NI Veristand/Custom Device API/Custom Device API.lvlib
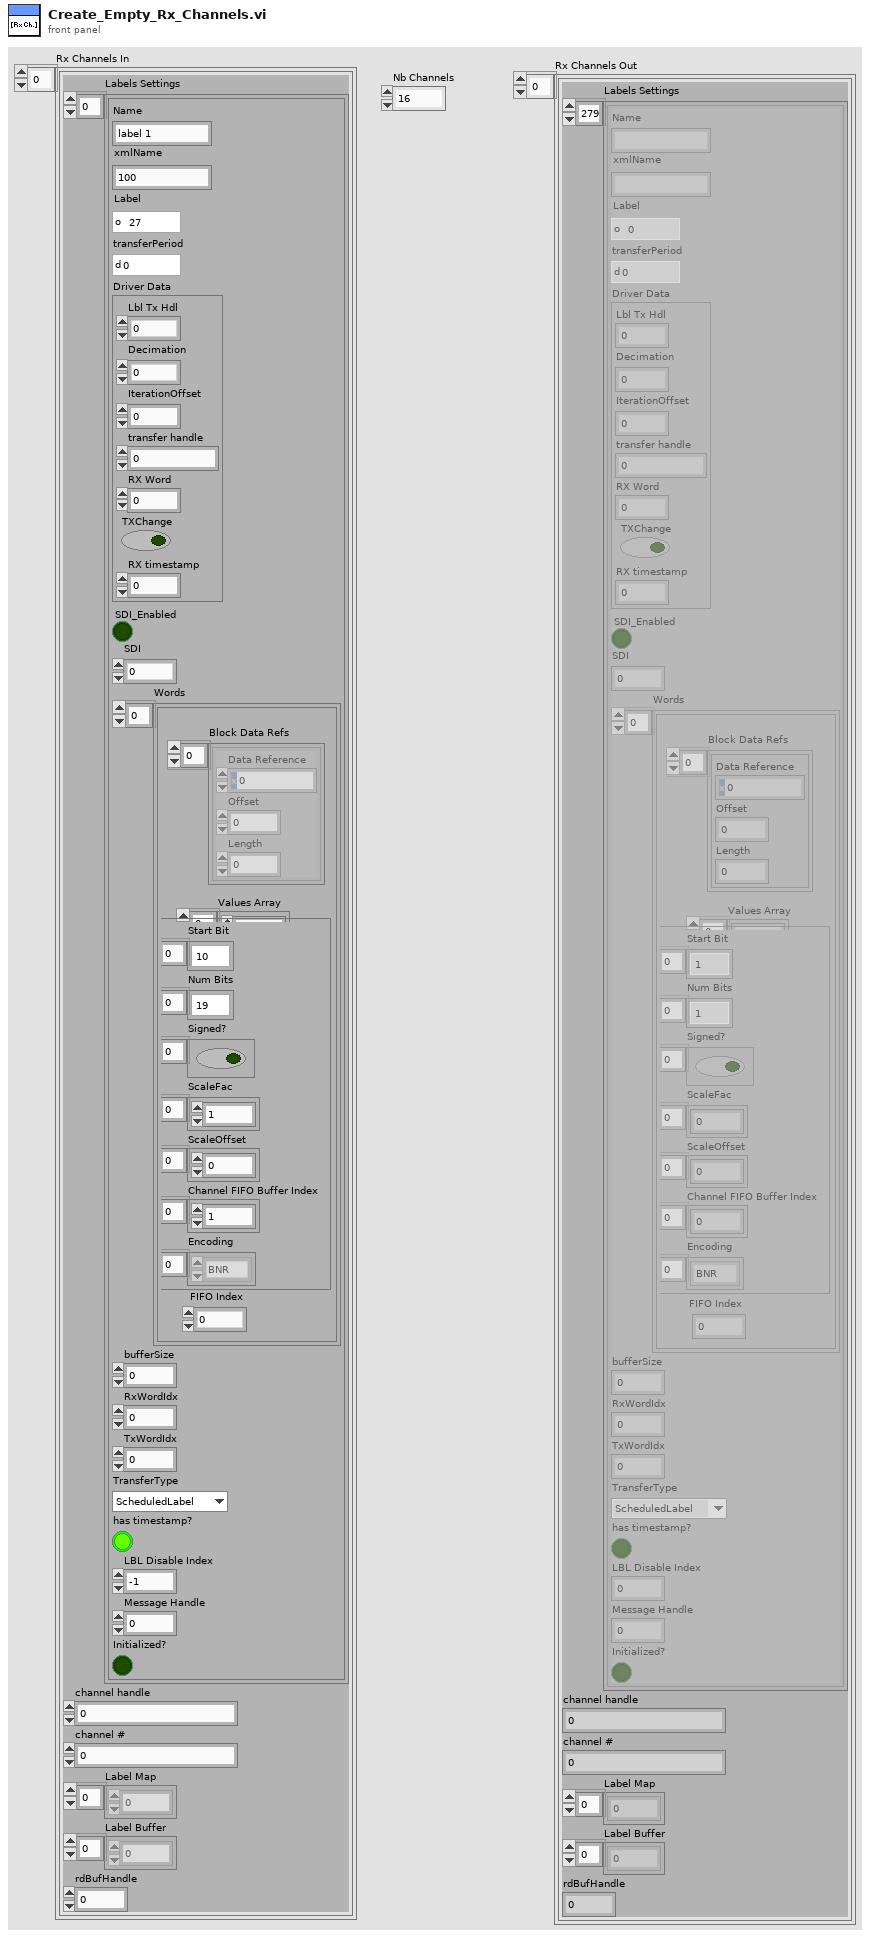
[diagram p1: front panel]
types:
  T1 = typedef "Ballard Arinc-429 Engine.lvlib/RT HW Channel.ctl" = cluster{"Labels Settings":T2[], "channel handle":u32, "channel #":u16, "Label Map":i32[], "Label Buffer":u32[], "rdBufHandle":u32}
  T2 = typedef "Ballard Arinc-429 Engine.lvlib/RT Label Settings.ctl" = cluster{"Name":string, "xmlName":string, "Label":T3, "transferPeriod":T4, "Driver Data":T5, "SDI_Enabled":bool, "SDI":u8, "Words":T6[], "bufferSize":u32, "RxWordIdx":i32, "TxWordIdx":i32, "TransferType":T12, "has timestamp?":bool, "LBL Disable Index":i32, "Message Handle":u64, "Initialized?":bool}
  T3 = typedef "Ballard Arinc-429 Shared.lvlib/Label.ctl" = u8
  T4 = typedef "Ballard Arinc-429 Shared.lvlib/transferPeriod.ctl" = u32
  T5 = typedef "Ballard Arinc-429 Engine.lvlib/Driver Data.ctl" = cluster{"Lbl Tx Hdl":u32, "Decimation":i32, "IterationOffset":i32, "transfer handle":u32, "RX Word":u32, "TXChange":bool, "RX timestamp":dbl}
  T6 = typedef "Ballard Arinc-429 Engine.lvlib/RT Word Settings.ctl" = cluster{"Block Data Refs":T7[], "Values Array":dbl[], "Length":i32, "FIFO Index":i32, "Param Setting":T9}
  T7 = typedef "Custom Device API.lvlib/Block Data Reference.ctl" = cluster{"Data Reference":T8, "Offset":u64, "Length":u64}
  T8 = typedef "Custom Device API.lvlib/Data Reference.ctl" = i32
  T9 = typedef "Ballard Arinc-429 Engine.lvlib/RT Param Setting.ctl" = cluster{"Start Bit":T10[], "Num Bits":T11[], "Signed?":bool[], "ScaleFac":dbl[], "ScaleOffset":dbl[], "Channel FIFO Buffer Index":i32[], "Encoding":enum16{"BNR", "BCD", "Discrete"}[]}
  T10 = typedef "Ballard Arinc-429 Shared.lvlib/Start Bit.ctl" = i32
  T11 = typedef "Ballard Arinc-429 Shared.lvlib/Number of Bits.ctl" = i32
  T12 = typedef "Ballard Arinc-429 Shared.lvlib/TransferType.ctl" = enum16{"ScheduledLabel", "Acyclic", "Block", "Strobe"}
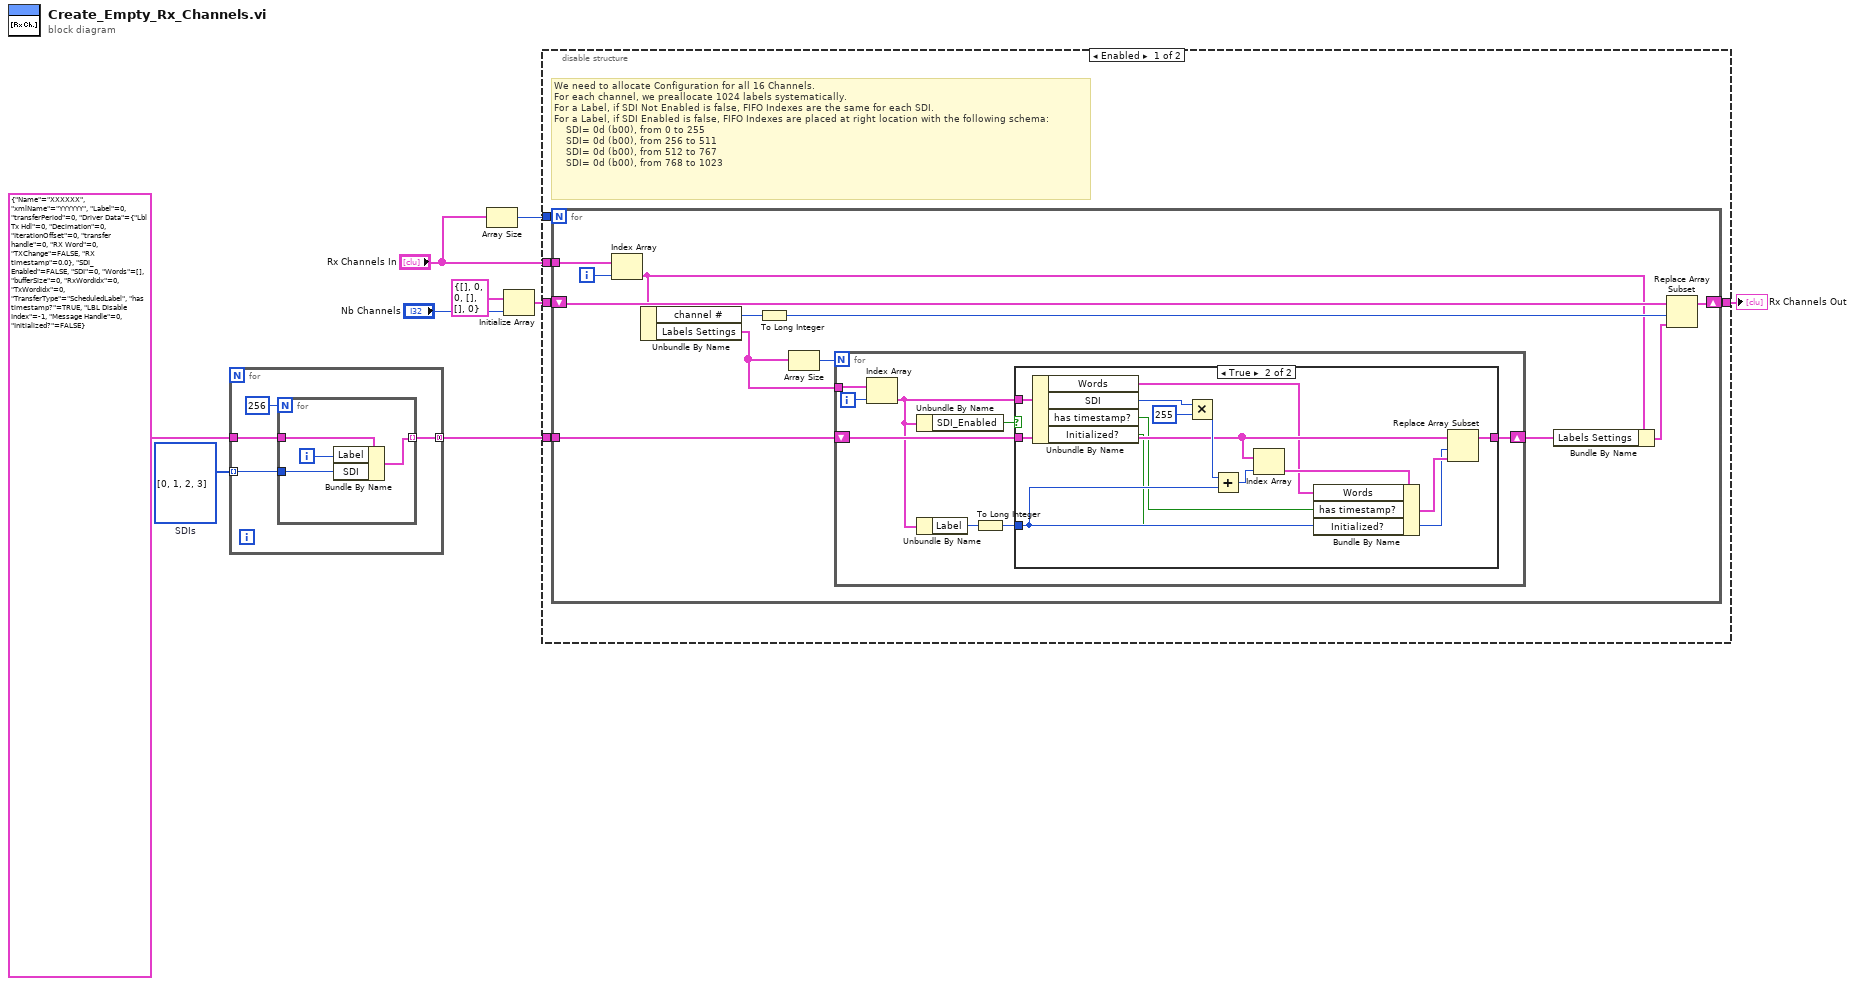
[diagram p0: block diagram]
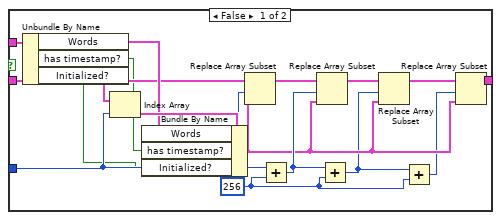
[diagram p2: hidden frame]
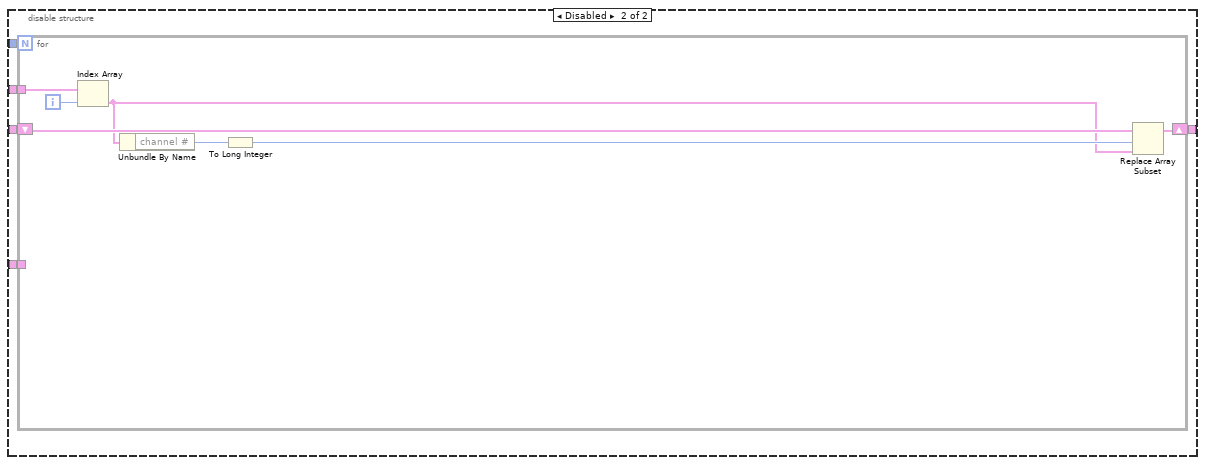
[diagram p3: hidden frame]
diagram:
  w2 = u8[] [0, 1, 2, 3]  # SDIs
  n1 = for {
    tunnel: T2 {"Name"="XXXXXX", "xmlName"="YYYYYY", "Label"=0, "transferPeriod"=0, "Driver Data"={"Lbl Tx Hdl"=0, "Decimation"=0, "IterationOffset"=0, "transfer handle"=0, "RX Word"=0, "TXChange"=FALSE, "RX timestamp"=0.0}, "SDI_Enabled"=FALSE, "SDI"=0, "Words"=[], "bufferSize"=0, "RxWordIdx"=0, "TxWordIdx"=0, "TransferType"=enum."ScheduledLabel", "has timestamp?"=TRUE, "LBL Disable Index"=-1, "Message Handle"=0, "Initialized?"=FALSE} ("Label Settings") -> [w12]
    tunnel: [w11] -> w1 mode=concatenating
    tunnel: w2 -> [w10] mode=indexing
    n2 = for {
      N: 256 -> [_]
      tunnel: w12 -> [w17]
      tunnel: [w15] -> w11 mode=indexing
      tunnel: w10 -> [w14]
      i -> [w16]
      n3 = Bundle By Name(cluster=w17, "Label"=w16, "SDI"=w14) -> (w15:T2)
    }
  }
  n4 = Array Size(array="Rx Channels In") -> (size(s)=w5:i32)
  n5 = Initialize Array(T1 {"Labels Settings"=[], "channel handle"=0, "channel #"=0, "Label Map"=[], "Label Buffer"=[], "rdBufHandle"=0} ("HW Channel"), "Nb Channels") -> (w7:T1[])
  n6 = disable-structure shown="Enabled" {
    disable-tunnel: w7 -> [w22 w76]
    disable-tunnel: [w21 w75] -> w6
    disable-tunnel: w5 -> [w20 w74]
    disable-tunnel: "Rx Channels In" -> [w19 w73]
    disable-tunnel: w1 -> [w18 w72]
    frame Enabled {
      # "We need to allocate Configuration for all 16 Channels.\nFor each channel, we preallocate 1024 labels systematically.\nFor a Label, if SDI Not Enabled is false, FIFO Indexes are the same for each SDI.\nFor a Label, if SDI Enabled is false, FIFO Indexes are placed at right location with the following schema:\n    SDI= 0d (b00), from 0 to 255\n    SDI= 0d (b00), from 256 to 511\n    SDI= 0d (b00), from 512 to 767\n    SDI= 0d (b00), from 768 to 1023"
      n7 = for {
        N: w20 -> [_]
        shift-right: [w32] -> w21
        shift-left: w22 -> [w33]
        tunnel: w19 -> [w31]
        tunnel: w18 -> [w28]
        i -> [w34]
        n8 = Index Array(array=w31, index=w34) -> (element=w25:T1)
        n9 = Unbundle By Name(w25) -> ("channel #"=w30:u16, "Labels Settings"=w27:T2[])
        n10 = To Long Integer(number=w30) -> (32bit integer=w29:i32)
        n11 = Array Size(array=w27) -> (size(s)=w26:i32)
        n12 = for {
          N: w26 -> [_]
          tunnel: w27 -> [w40]
          shift-right: [w35] -> w24
          shift-left: w28 -> [w41]
          i -> [w39]
          n13 = Index Array(array=w40, index=w39) -> (element=w38:T2)
          n14 = Unbundle By Name(w38) -> ("SDI_Enabled"=w42:bool)
          n15 = Unbundle By Name(w38) -> ("Label"=w37:T3)
          n16 = To Long Integer(number=w37) -> (32bit integer=w36:i32)
          n17 = case shown="True" w42 {
            tunnel: w41 -> [w55 w66]
            tunnel: w38 -> [w58 w71]
            tunnel: w36 -> [w54 w62]
            tunnel: [w45 w61] -> w35
            frame False {
              w48 = 256 ("y")
              n18 = Unbundle By Name(w58) -> ("Words"=w56:T6[], "has timestamp?"=w44:bool, "Initialized?"=w43:bool)
              n19 = Index Array(array=w55, index=w54) -> (element=w57:T2)
              n20 = Bundle By Name(cluster=w57, "Words"=w56, "has timestamp?"=w44, "Initialized?"=w43) -> (w50:T2)
              n21 = Replace Array Subset(array=w55, new element=w50, index=w54) -> (w53:T2[])
              n22 = Add(x=w54, y=w48) -> (x+y=w52:i32)
              n23 = Replace Array Subset(array=w53, new element=w50, index=w52) -> (w51:T2[])
              n24 = Add(x=w52, y=w48) -> (x+y=w49:i32)
              n25 = Replace Array Subset(array=w51, new element=w50, index=w49) -> (w46:T2[])
              n26 = Add(x=w49, y=w48) -> (x+y=w47:i32)
              n27 = Replace Array Subset(array=w46, new element=w50, index=w47) -> (w45:T2[])
            }
            frame True {
              n28 = Unbundle By Name(w71) -> ("Words"=w63:T6[], "SDI"=w70:u8, "has timestamp?"=w60:bool, "Initialized?"=w59:bool)
              n29 = Multiply(x=w70, y=255) -> (x*y=w68:i32)
              n30 = Add(x=w68, y=w62) -> (x+y=w67:i32)
              n31 = Index Array(array=w66, index=w67) -> (element=w65:T2)
              n32 = Bundle By Name(cluster=w65, "Words"=w63, "has timestamp?"=w60, "Initialized?"=w59) -> (w64:T2)
              n33 = Replace Array Subset(array=w66, new element=w64, index=w62) -> (w61:T2[])
            }
          }
        }
        n34 = Bundle By Name(cluster=w25, "Labels Settings"=w24) -> (w23:T1)
        n35 = Replace Array Subset(array=w33, new element=w23, index=w29) -> (w32:T1[])
      }
    }
    frame Disabled {
      n36 = for {
        N: w74 -> [_]
        shift-right: [w81] -> w75
        shift-left: w76 -> [w82]
        tunnel: w73 -> [w80]
        tunnel: w72 -> [_]
        i -> [w83]
        n37 = Index Array(array=w80, index=w83) -> (element=w77:T1)
        n38 = Unbundle By Name(w77) -> ("channel #"=w79:u16)
        n39 = To Long Integer(number=w79) -> (32bit integer=w78:i32)
        n40 = Replace Array Subset(array=w82, new element=w77, index=w78) -> (w81:T1[])
      }
    }
  }
  "Rx Channels Out" <- w6
